vi "calcRigidBodyH.vi"(8 "error in (no error)":errorcluster, 10 "Rigid Body Stroke File":string="rbStroke.txt", 11 "OptCtrl in":refnum<class "OptCtrl.lvclass">) -> (0 "error out":errorcluster, 2 "Authority (1 um)":dbl[](array[numeric]), 3 "OptCtrl out":refnum<class "OptCtrl.lvclass">)   [LabVIEW 2016, in "OptCtrl.lvclass"]
doc: "Calculate the distribution of control authority of rigid body."
uses:
  OptCtrl.lvclass
  OptCtrl.lvclass/OptCtrl.ctl
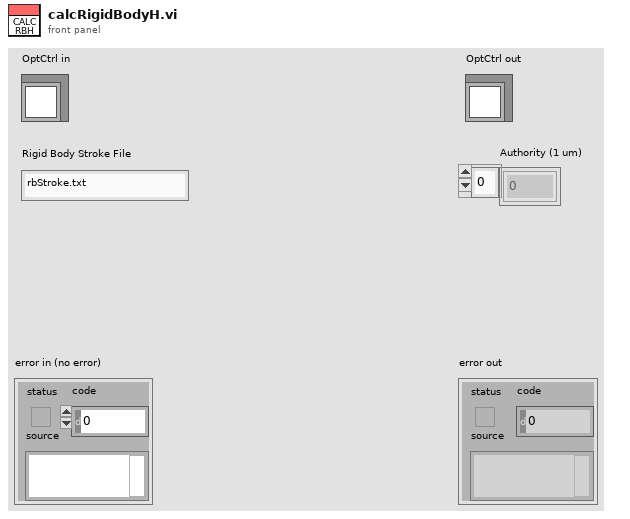
[diagram p1: front panel]
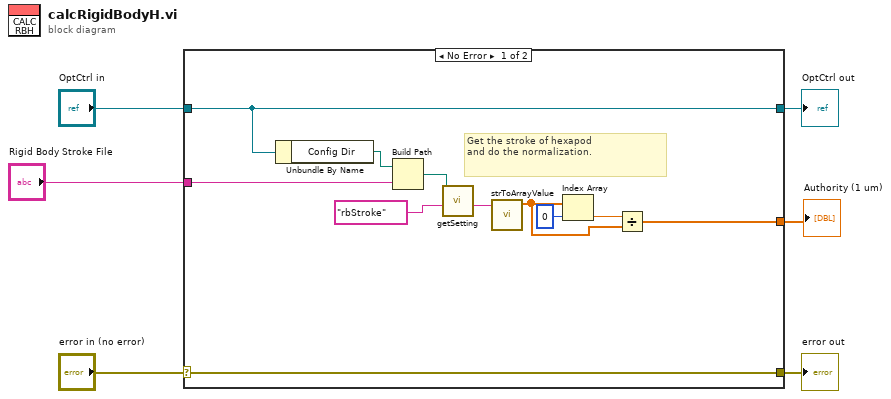
[diagram p0: block diagram]
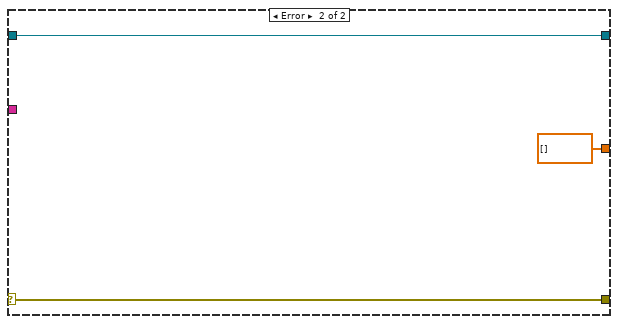
[diagram p2: hidden frame]
diagram:
  n1 = case shown="No Error" "error in (no error)" {
    selector: "error in (no error)" -> [w17 w20]
    tunnel: [w17 w20] -> w5
    tunnel: [w9 w19] -> w3
    tunnel: "OptCtrl in" -> [w9 w19]
    tunnel: "Rigid Body Stroke File" -> [w8 _]
    tunnel: [w7 dbl[] []] -> w1
    frame No Error {
      # "Get the stroke of hexapod \nand do the normalization."
      n2 = Unbundle By Name(w9) -> ("Config Dir"=w16:path)
      n3 = Build Path(base path=w16, name or relative path=w8) -> (appended path=w15:path)
      n4 = call "getSetting.vi"("Parameter"="rbStroke", "Path"=w15) -> ("Value"=w13:string)  [unwired: 8 in, 1 out]
      n5 = call "strToArrayValue.vi"("String"=w13) -> ("Array"=w10:dbl[])  [unwired: 10 in]
      n6 = Index Array(array=w10, index=0) -> (element=w11:dbl)
      n7 = Divide(x=w11, y=w10) -> (x/y=w7:dbl[])
    }
    frame Error {
    }
  }
  "error out" <- w5
  "OptCtrl out" <- w3
  "Authority (1 um)" <- w1
